vi "Global tdms reference.vi"() -> ()   [LabVIEW 2016]
panel:
  out "PV tdms file out":refnum<k34>
  out "Switch tdms file out":refnum<k34>
  out "Batt tdms file out":refnum<k34>
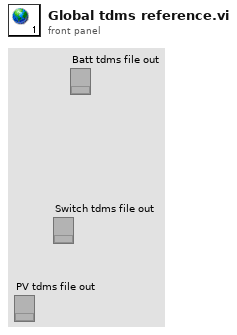
[diagram p1: front panel]
diagram:
